vi "SetAmplitudeModulation.vi"(8 "b_am":fxp<+/-,16,2>, 9 "a_am":fxp<+/-,16,2>, 10 "Am freq [kHz]":dbl=10.0, 11 "scope in":T1) -> (3 "scope out":T1)   [LabVIEW 2013]
uses:
  controls/scope_params_5782.ctl
  Utilities/Ticker/Ticker.lvclass
  Communication/Driver/RemoteConnection/RemoteConnection.lvclass
  Scope/controls/ScopeMode.ctl
  Config/FPGAref_5782.ctl
  FPGA/DataMode.ctl
  controls/5782_trigger_type.ctl
  <vilib>/rvi/interface/common/niFpgaWaitOnOcc.vi
  <vilib>/Utility/error.llb/Error Cluster From Error Code.vi
  <vilib>/rvi/errors/niLvFpgaAdjustHostInterfaceError.vi
  <vilib>/rvi/interface/nirviReadWriteControl/nirviReadWriteControl.xnode
  NiFpgaLv.dll
  <vilib>/rvi/interface/Simulation/niFpgaSimulationCallBeginRW.vi
panel:
  out "error out":errorcluster
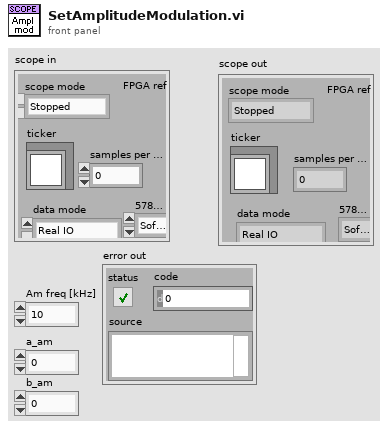
[diagram p1: front panel]
types:
  T1 = typedef "scope_params_5782.ctl" = cluster{"scope mode":T2, "ticker":refnum<class "Ticker.lvclass">, "samples per record":i32, "FPGA ref":T3, "data mode":T4, "5782 Trigger":T5, "Chart length":i32, "RemoteConnection":refnum<class "RemoteConnection.lvclass">}
  T2 = typedef "ScopeMode.ctl" = enum16{"Stopped", "Single", "Running", "Continuous"}
  T3 = typedef "FPGAref_5782.ctl" = refnum<k20>
  T4 = typedef "DataMode.ctl" = enum16{"Real IO", "Simulated"}
  T5 = typedef "5782_trigger_type.ctl" = enum16{"Software", "Trigger input"}
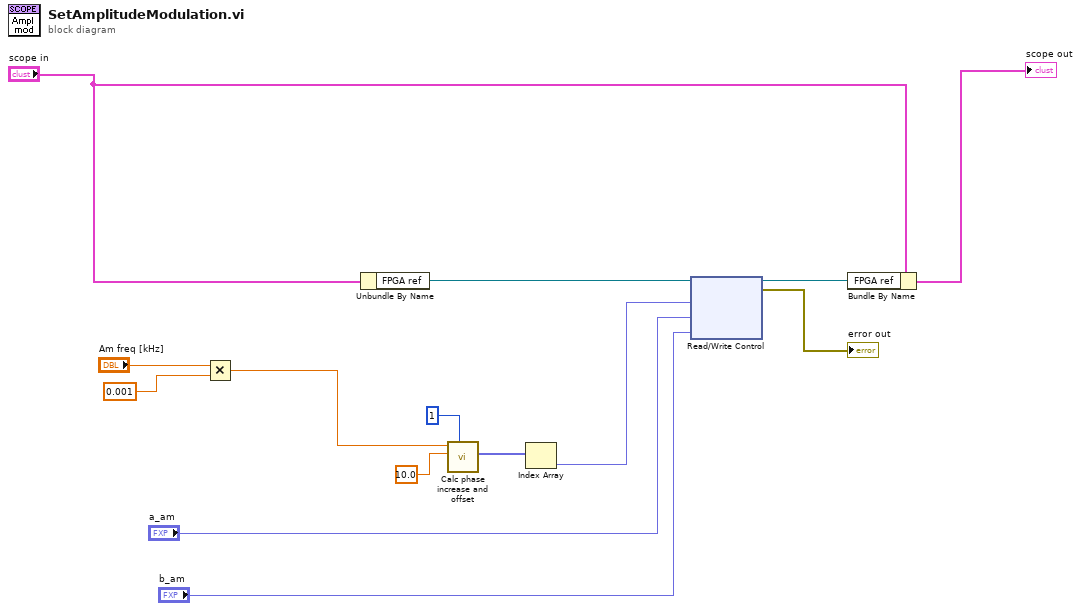
[diagram p0: block diagram]
diagram:
  n1 = Multiply(x="Am freq [kHz]", y=0.001) -> (x*y=w6:dbl)
  n2 = Unbundle By Name("scope in") -> ("FPGA ref"=w14:T3)
  n3 = call "Calc phase increase and offset.vi"("# of DDS"=1, "fclk (MHz)"=10.0, "f_generated (MHz)"=w6) -> ("Phase out"=w8:fxp<+,64,64>[])  [unwired: 6 in, 2 out]
  n4 = Index Array(array=w8) -> (element=w7:fxp<+,64,64>)  [unwired: 1 in]
  n5 = xnode "Read/Write Control"("FPGA VI Reference In"=w14, "AM phase"=w7, "a_am"="a_am", "b_am"="b_am") -> ("FPGA VI Reference Out"=w13:T3, "error out"=→"error out":errorcluster)  [unwired: 1 in]
  n6 = Bundle By Name(cluster="scope in", "FPGA ref"=w13) -> (→"scope out":T1)
